vi "MakeWhitePlot.vi"(7 "Canvas":refnum<vi>, 8 "# harmonics":i32=40, 9 "# freq":i32=48, 10 "Bounds":T1, 11 "Complex In":cluster{dbl, "df":dbl, cdb[]}[](array[cluster])) -> (3 "Graph":picture)   [LabVIEW 2022 SP3]
uses:
  <vilib>/Utility/miscctls.llb/LVBoundsTypeDef.ctl
  Perspective/subs/Perspective_Globals.vi
panel:
  out "TRF":cluster{dbl, "df":dbl, dbl[]}(graph)={199.951171875, "df"=0.732421875, array[13381 elements]}
  out "2D Plot":dbl[][](graph)=[[nan, 20.049987226429913, 25.054902961250857, 29.445158043811198, 34.46385501795731, 44.780627225419565, 51.406191185965646, 49.67631609372249, 40.709611963732584, 38.92269108407762, 40.35029451326228, 33.055745098571954, 41.52467260523725, 39.21617102292643, 15.173302135246772, 40.695109109084115, 42.444899082336, 56.77593405896198, 51.382201329207334, 43.21477455890306, 50.80370011373546, 35.98612449368547, 47.77204513443894, 30.857881410259274, 46.643671439889445, 47.49403661581599, -1.4346363375750995, 19.0211768965106, 45.28695989710588, 40.69907700152897, 46.376353342172045, 39.045432783467874, 48.20425730785347, 35.99159002094946, 35.20324613314526, 51.91563451765467, 18.854037759092634, 37.28439063047342, -19.57168106597702, 25.22610299025189, 29.263013635587455, 30.82063676591259, 33.55395737125039, 18.19981181386353, 24.102157288646847, 39.34971755858826, 22.241809662116708, 68.52224965159985], [54.26627490024298, 47.12526752661166, 56.85500723817575, 36.55833093424573, 38.634265924869595, 51.93988341853376, 45.638032395871505, 66.45923338856223, 48.341086236955675, 44.73549896684294, 82.8746731094306, 36.13504669577988, 32.4985458705831, 38.46882120330299, 25.627379738354886, 38.640118352136994, 69.51016913200667, 47.08441844740895, 43.538098543664844, 37.74770538349388, 2.607749244145145, 35.43065545900197, 48.78584596653637, 44.50117153673708, 47.18149466094815, 37.167565780443084, -11.290057999008061, 38.82305284871714, 34.622338104545236, 45.77689163136356, 27.988762535569126, 35.05040002787151, 46.39143083402964, 41.744798474139316, 32.89651926775419, 62.34466322011301, 39.44356696797309, 46.6442728756223, -10.828073640077598, 26.81232522566393, 48.71727144928745, 32.03610040569839, 72.79095309960253, 36.67913423432094, 48.058266713190754, nan, nan, nan], [53.04185758812355, 84.71388448770111, 17.51080377410179, 40.44091855599027, 39.91331658353087, 28.362665427675545, 55.229556863313356, 56.42371074485528, 47.76931799964777, 39.97049168305633, 57.15726261780386, 37.542352295940155, 44.21162796738528, 17.48325982608004, 40.43782874904303, 38.742739205630784, 46.032627402046785, 20.05630274646011, 45.78665416858822, 35.24520049827762, 39.158716639789034, 11.924005690223789, 29.897529283546916, 33.60264045829483, 31.392790303731708, 19.506700819440113, -9.215795080095525, 50.42813350565264, 32.59479614372741, 31.01757424069985, 42.71237559822864, 51.983617982184924, 34.35731157695301, 42.627623260331376, 19.10147623463881, 54.50616438544329, 18.296402637224976, 58.61753732987064, nan, nan, nan, nan, nan, nan, nan, nan, nan, nan], [39.51596652723599, 29.184271442763787, 16.957827346664814, 37.67653983236719, 63.59782300125275, 48.322834414258296, 40.39060448678149, 38.07851466585304, 52.219678596166396, 61.51482106592874, 46.8634576004301, 37.06553982367735, 38.09179565041872, 11.208063972191031, 54.731123202538576, 29.039234290370757, 34.051601948841004, 41.1260225901982, 52.08899147984912, 28.05180790327435, 34.07973803463468, 42.3996411700281, 20.192703080247497, 56.168607595418976, 33.25620455392025, 39.61259618090587, 1.6416847986202243, 24.841476380656804, 37.55245428572219, 27.459839855335257, 66.77063240632266, 36.5729389128255, 41.814287416945945, nan, nan, nan, nan, nan, nan, nan, nan, nan, nan, nan, nan, nan, nan, nan], [48.16850062624863, 42.24542108686359, 44.340073178907026, 3.901363084528417, 42.347676492963295, 41.98102702804944, 32.095730941153256, 7.619084984059836, 32.35066397625168, 32.29142786493228, 40.21124807070387, 14.63732432854075, 64.87319042636963, 3.8937001997797758, 42.35230450100133, 14.130476829463692, 28.642057668910525, 38.68345012614008, 40.520552066845205, 52.826865227382584, 27.4036034714791, 73.37393650330726, 10.947826509906172, 39.440434175724384, 31.785624530969287, 39.726239419396016, 27.00365963632292, 17.381561857680012, 36.93147689751727, nan, nan, nan, nan, nan, nan, nan, nan, nan, nan, nan, nan, nan, nan, nan, nan, nan, nan, nan], [35.60423156346238, 46.08009523979531, 36.87411957248013, 43.245886090198724, 41.3473179130062, 26.344792341973875, 41.08933756077456, 27.303763144444684, 32.28100773510765, 34.38861713258833, 31.00322874795537, 55.966772111396814, 33.80384369988236, 22.921989435884473, 8.945740357752978, 42.39269732229077, 33.87217699897191, 33.14532562541018, 33.524294370197566, 44.041506495823185, 37.757502066680686, 41.939614181516674, 8.546073278104322, 48.000016608061514, 35.00765134648421, 51.85386377302325, nan, nan, nan, nan, nan, nan, nan, nan, nan, nan, nan, nan, nan, nan, nan, nan, nan, nan, nan, nan, nan, nan], [32.61310636745673, 38.97527846530624, 35.641622198785086, 36.36206724043218, 27.795949148894337, 54.187637574190326, 36.401734072540044, 30.917571343879366, 37.20179247250486, 27.793291744454113, 25.775060428523826, 10.666225801452157, 38.49962709844564, 11.781027471364073, 13.761017548356374, 42.53126220573978, 35.128829087408405, 40.161072813389424, 41.09343386515138, 35.9780075897034, 17.001024691654287, 42.92404272966259, 26.64675831650957, nan, nan, nan, nan, nan, nan, nan, nan, nan, nan, nan, nan, nan, nan, nan, nan, nan, nan, nan, nan, nan, nan, nan, nan, nan], [29.681571025848356, 42.60929144128346, 48.67052729500847, 58.6607561868737, 33.95354038216709, 41.11614535668331, 47.65431912163869, -11.009770350280277, 36.94947500875874, 39.83841719056124, 31.381560080516877, 52.500057048302736, 38.174458325750436, 20.80842003831775, 12.283677007960899, 35.16227099829001, 59.770944975043896, 21.937359659167246, 60.53209358540707, 36.682904986845664, 39.7581113435772, nan, nan, nan, nan, nan, nan, nan, nan, nan, nan, nan, nan, nan, nan, nan, nan, nan, nan, nan, nan, nan, nan, nan, nan, nan, nan, nan], [40.464054607466934, 37.58597485171173, 39.87038706581357, 51.19267039727471, 37.67639985297179, 23.13937723997912, 37.55595835553924, 42.4209222579333, 42.27910760517511, 30.522265980669758, 26.136408931304445, -2.9872106006803496, 31.322538117444275, 2.9044348449634656, 3.5797530867064515, 50.092277015634636, 38.50977087060315, 47.533818499292835, 35.62939006713031, nan, nan, nan, nan, nan, nan, nan, nan, nan, nan, nan, nan, nan, nan, nan, nan, nan, nan, nan, nan, nan, nan, nan, nan, nan, nan, nan, nan, nan], [58.5659239452997, 26.982848813621306, 36.31906856692317, 16.66678219935681, 49.49109923197512, 40.11411668922503, 37.75341628139453, 48.30992190831356, 49.081010121114915, 61.181425385472934, 22.430170217674966, 48.6155340973561, 32.675460627661636, 13.916675441379617, 21.021585447450946, 49.25166283256742, 62.27105544588605, nan, nan, nan, nan, nan, nan, nan, nan, nan, nan, nan, nan, nan, nan, nan, nan, nan, nan, nan, nan, nan, nan, nan, nan, nan, nan, nan, nan, nan, nan, nan], [54.412382522142494, 36.137207842053776, 2.764148858981666, 46.372145605984485, 37.243085887419376, 34.537737023825855, 55.257207308976035, 51.464533050016435, 39.80085824725523, 44.11810710124637, 34.10663843132296, 5.979096794947166, 25.782557120064702, 30.561510305365577, 40.94721364933057, nan, nan, nan, nan, nan, nan, nan, nan, nan, nan, nan, nan, nan, nan, nan, nan, nan, nan, nan, nan, nan, nan, nan, nan, nan, nan, nan, nan, nan, nan, nan, nan, nan], [31.369910198236113, 37.07152928092298, 10.648427094010238, 40.65058675099788, 23.51231403437172, 27.206691169768323, 36.277462506216686, 34.08022467450811, 35.763375497264654, 29.232268970303785, 23.380681094116376, 44.186129447967446, 35.05238954844841, 50.27126063942963, nan, nan, nan, nan, nan, nan, nan, nan, nan, nan, nan, nan, nan, nan, nan, nan, nan, nan, nan, nan, nan, nan, nan, nan, nan, nan, nan, nan, nan, nan, nan, nan, nan, nan], [47.82026138668182, 33.43812207351204, 25.299758140785883, -0.1217403502671347, 22.16453525325594, 48.48725544404082, 42.08447575914906, 19.62567783478579, 38.80170108501365, 40.192102073325636, 33.03273363219364, 36.03429599678489, 28.409628306750335, nan, nan, nan, nan, nan, nan, nan, nan, nan, nan, nan, nan, nan, nan, nan, nan, nan, nan, nan, nan, nan, nan, nan, nan, nan, nan, nan, nan, nan, nan, nan, nan, nan, nan, nan], [38.74276193034642, 51.348432885653914, 32.25091267120466, 38.33577783712102, 29.752691953524675, 38.079351040376174, 38.87949376223, 0.26530157389657355, 29.509618670886084, 40.33082643082275, 34.24093489901787, nan, nan, nan, nan, nan, nan, nan, nan, nan, nan, nan, nan, nan, nan, nan, nan, nan, nan, nan, nan, nan, nan, nan, nan, nan, nan, nan, nan, nan, nan, nan, nan, nan, nan, nan, nan, nan], [38.005167377161804, 31.69088276912158, 52.845640027356204, 35.852538445709634, 43.1225994596063, 37.243651148967345, 29.029508255433182, 9.006139857266586, 38.32944523498376, 36.834360308878054, nan, nan, nan, nan, nan, nan, nan, nan, nan, nan, nan, nan, nan, nan, nan, nan, nan, nan, nan, nan, nan, nan, nan, nan, nan, nan, nan, nan, nan, nan, nan, nan, nan, nan, nan, nan, nan, nan], [35.90269660816785, 39.364578709379494, 39.55419749173399, 29.35326642077404, 53.69867614237862, 31.967502560639367, 54.7193336975603, 30.88778141801589, 39.34981484445568, nan, nan, nan, nan, nan, nan, nan, nan, nan, nan, nan, nan, nan, nan, nan, nan, nan, nan, nan, nan, nan, nan, nan, nan, nan, nan, nan, nan, nan, nan, nan, nan, nan, nan, nan, nan, nan, nan, nan], [36.30638411087302, 25.09057920682725, 45.46164717529554, 49.768103526439276, 23.289405968677816, 49.15198590837125, 35.1560324577208, 42.864683043159424, nan, nan, nan, nan, nan, nan, nan, nan, nan, nan, nan, nan, nan, nan, nan, nan, nan, nan, nan, nan, nan, nan, nan, nan, nan, nan, nan, nan, nan, nan, nan, nan, nan, nan, nan, nan, nan, nan, nan, nan], [31.462436582201292, 30.362788351721534, 36.81834627839507, 44.09040502089316, 33.57068005060175, 32.74557557265104, 39.515790233414656, nan, nan, nan, nan, nan, nan, nan, nan, nan, nan, nan, nan, nan, nan, nan, nan, nan, nan, nan, nan, nan, nan, nan, nan, nan, nan, nan, nan, nan, nan, nan, nan, nan, nan, nan, nan, nan, nan, nan, nan, nan], [34.58411077100862, 33.23559013285732, -5.662822029697699, 26.44794576028672, 35.487431815874324, 40.942138140629154, nan, nan, nan, nan, nan, nan, nan, nan, nan, nan, nan, nan, nan, nan, nan, nan, nan, nan, nan, nan, nan, nan, nan, nan, nan, nan, nan, nan, nan, nan, nan, nan, nan, nan, nan, nan, nan, nan, nan, nan, nan, nan], [34.61465926871371, 17.18392844569568, 13.031570274998831, 43.78480234185166, 56.1573881112846, nan, nan, nan, nan, nan, nan, nan, nan, nan, nan, nan, nan, nan, nan, nan, nan, nan, nan, nan, nan, nan, nan, nan, nan, nan, nan, nan, nan, nan, nan, nan, nan, nan, nan, nan, nan, nan, nan, nan, nan, nan, nan, nan], [29.186029345513607, 47.978737915500574, 17.360000383750858, 12.786831883362723, nan, nan, nan, nan, nan, nan, nan, nan, nan, nan, nan, nan, nan, nan, nan, nan, nan, nan, nan, nan, nan, nan, nan, nan, nan, nan, nan, nan, nan, nan, nan, nan, nan, nan, nan, nan, nan, nan, nan, nan, nan, nan, nan, nan], [25.72159338389789, 36.84666611970028, 34.76691669928632, nan, nan, nan, nan, nan, nan, nan, nan, nan, nan, nan, nan, nan, nan, nan, nan, nan, nan, nan, nan, nan, nan, nan, nan, nan, nan, nan, nan, nan, nan, nan, nan, nan, nan, nan, nan, nan, nan, nan, nan, nan, nan, nan, nan, nan], [27.424976418713154, 38.48369817799687, 50.658137928834435, nan, nan, nan, nan, nan, nan, nan, nan, nan, nan, nan, nan, nan, nan, nan, nan, nan, nan, nan, nan, nan, nan, nan, nan, nan, nan, nan, nan, nan, nan, nan, nan, nan, nan, nan, nan, nan, nan, nan, nan, nan, nan, nan, nan, nan], [34.75082504002703, 44.286747839093266, nan, nan, nan, nan, nan, nan, nan, nan, nan, nan, nan, nan, nan, nan, nan, nan, nan, nan, nan, nan, nan, nan, nan, nan, nan, nan, nan, nan, nan, nan, nan, nan, nan, nan, nan, nan, nan, nan, nan, nan, nan, nan, nan, nan, nan, nan], [35.40073024186071, nan, nan, nan, nan, nan, nan, nan, nan, nan, nan, nan, nan, nan, nan, nan, nan, nan, nan, nan, nan, nan, nan, nan, nan, nan, nan, nan, nan, nan, nan, nan, nan, nan, nan, nan, nan, nan, nan, nan, nan, nan, nan, nan, nan, nan, nan, nan], [28.955349958389448, nan, nan, nan, nan, nan, nan, nan, nan, nan, nan, nan, nan, nan, nan, nan, nan, nan, nan, nan, nan, nan, nan, nan, nan, nan, nan, nan, nan, nan, nan, nan, nan, nan, nan, nan, nan, nan, nan, nan, nan, nan, nan, nan, nan, nan, nan, nan], [nan, nan, nan, nan, nan, nan, nan, nan, nan, nan, nan, nan, nan, nan, nan, nan, nan, nan, nan, nan, nan, nan, nan, nan, nan, nan, nan, nan, nan, nan, nan, nan, nan, nan, nan, nan, nan, nan, nan, nan, nan, nan, nan, nan, nan, nan, nan, nan], [nan, nan, nan, nan, nan, nan, nan, nan, nan, nan, nan, nan, nan, nan, nan, nan, nan, nan, nan, nan, nan, nan, nan, nan, nan, nan, nan, nan, nan, nan, nan, nan, nan, nan, nan, nan, nan, nan, nan, nan, nan, nan, nan, nan, nan, nan, nan, nan], [nan, nan, nan, nan, nan, nan, nan, nan, nan, nan, nan, nan, nan, nan, nan, nan, nan, nan, nan, nan, nan, nan, nan, nan, nan, nan, nan, nan, nan, nan, nan, nan, nan, nan, nan, nan, nan, nan, nan, nan, nan, nan, nan, nan, nan, nan, nan, nan], [nan, nan, nan, nan, nan, nan, nan, nan, nan, nan, nan, nan, nan, nan, nan, nan, nan, nan, nan, nan, nan, nan, nan, nan, nan, nan, nan, nan, nan, nan, nan, nan, nan, nan, nan, nan, nan, nan, nan, nan, nan, nan, nan, nan, nan, nan, nan, nan], [nan, nan, nan, nan, nan, nan, nan, nan, nan, nan, nan, nan, nan, nan, nan, nan, nan, nan, nan, nan, nan, nan, nan, nan, nan, nan, nan, nan, nan, nan, nan, nan, nan, nan, nan, nan, nan, nan, nan, nan, nan, nan, nan, nan, nan, nan, nan, nan], [nan, nan, nan, nan, nan, nan, nan, nan, nan, nan, nan, nan, nan, nan, nan, nan, nan, nan, nan, nan, nan, nan, nan, nan, nan, nan, nan, nan, nan, nan, nan, nan, nan, nan, nan, nan, nan, nan, nan, nan, nan, nan, nan, nan, nan, nan, nan, nan], [nan, nan, nan, nan, nan, nan, nan, nan, nan, nan, nan, nan, nan, nan, nan, nan, nan, nan, nan, nan, nan, nan, nan, nan, nan, nan, nan, nan, nan, nan, nan, nan, nan, nan, nan, nan, nan, nan, nan, nan, nan, nan, nan, nan, nan, nan, nan, nan], [nan, nan, nan, nan, nan, nan, nan, nan, nan, nan, nan, nan, nan, nan, nan, nan, nan, nan, nan, nan, nan, nan, nan, nan, nan, nan, nan, nan, nan, nan, nan, nan, nan, nan, nan, nan, nan, nan, nan, nan, nan, nan, nan, nan, nan, nan, nan, nan], [nan, nan, nan, nan, nan, nan, nan, nan, nan, nan, nan, nan, nan, nan, nan, nan, nan, nan, nan, nan, nan, nan, nan, nan, nan, nan, nan, nan, nan, nan, nan, nan, nan, nan, nan, nan, nan, nan, nan, nan, nan, nan, nan, nan, nan, nan, nan, nan], [nan, nan, nan, nan, nan, nan, nan, nan, nan, nan, nan, nan, nan, nan, nan, nan, nan, nan, nan, nan, nan, nan, nan, nan, nan, nan, nan, nan, nan, nan, nan, nan, nan, nan, nan, nan, nan, nan, nan, nan, nan, nan, nan, nan, nan, nan, nan, nan], [nan, nan, nan, nan, nan, nan, nan, nan, nan, nan, nan, nan, nan, nan, nan, nan, nan, nan, nan, nan, nan, nan, nan, nan, nan, nan, nan, nan, nan, nan, nan, nan, nan, nan, nan, nan, nan, nan, nan, nan, nan, nan, nan, nan, nan, nan, nan, nan], [nan, nan, nan, nan, nan, nan, nan, nan, nan, nan, nan, nan, nan, nan, nan, nan, nan, nan, nan, nan, nan, nan, nan, nan, nan, nan, nan, nan, nan, nan, nan, nan, nan, nan, nan, nan, nan, nan, nan, nan, nan, nan, nan, nan, nan, nan, nan, nan], [nan, nan, nan, nan, nan, nan, nan, nan, nan, nan, nan, nan, nan, nan, nan, nan, nan, nan, nan, nan, nan, nan, nan, nan, nan, nan, nan, nan, nan, nan, nan, nan, nan, nan, nan, nan, nan, nan, nan, nan, nan, nan, nan, nan, nan, nan, nan, nan], [nan, nan, nan, nan, nan, nan, nan, nan, nan, nan, nan, nan, nan, nan, nan, nan, nan, nan, nan, nan, nan, nan, nan, nan, nan, nan, nan, nan, nan, nan, nan, nan, nan, nan, nan, nan, nan, nan, nan, nan, nan, nan, nan, nan, nan, nan, nan, nan]]
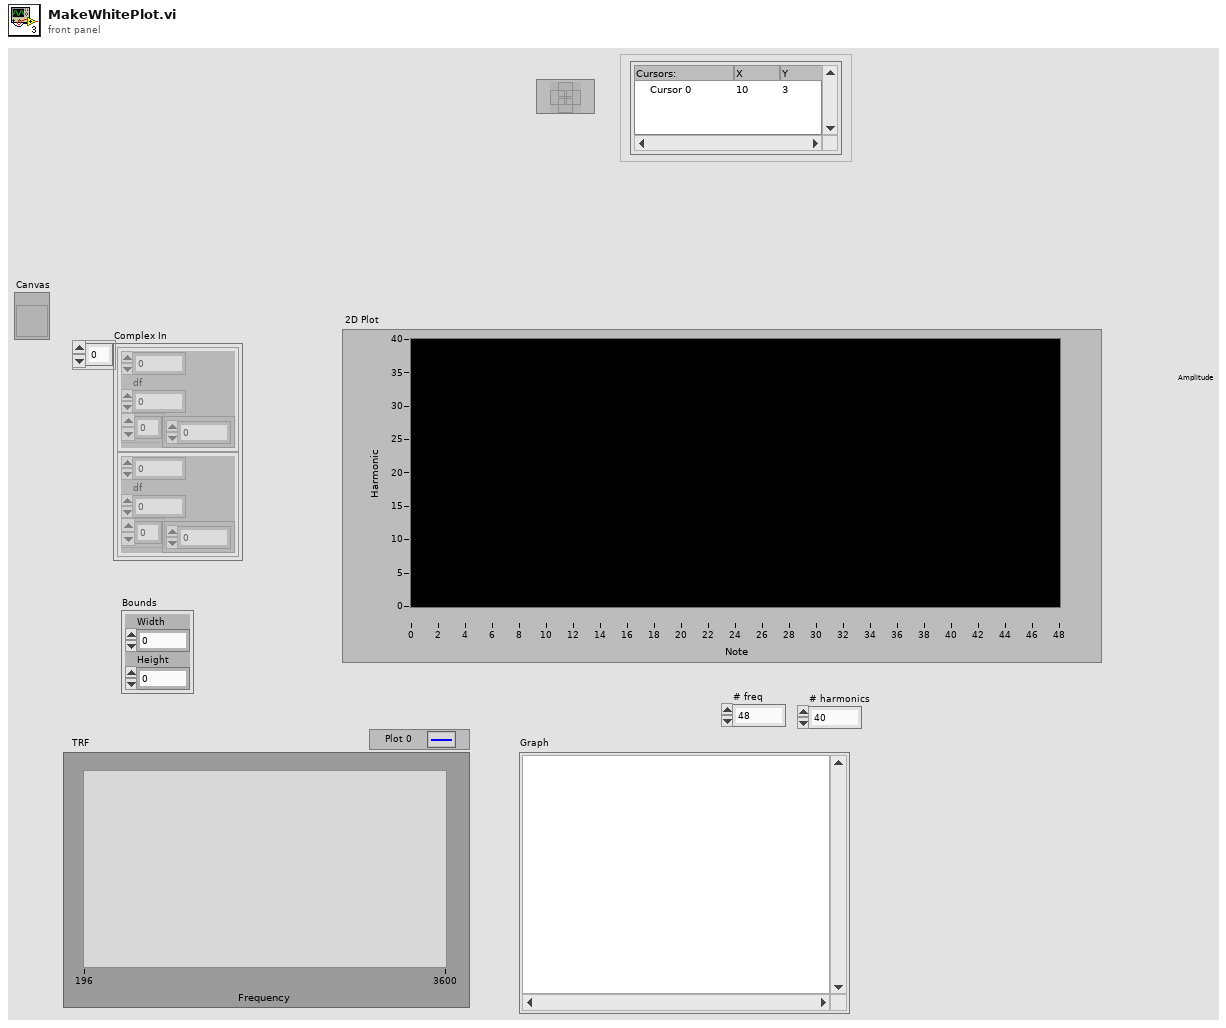
[diagram p1: front panel]
types:
  T1 = typedef "LVBoundsTypeDef.ctl" = cluster{"Width":u32, "Height":u32}
  T2 = enum16{"Sine Wave", "Triangle Wave", "Square Wave", "Sawtooth Wave"}
  T3 = cluster{"Notes":string, "format string":string}[]
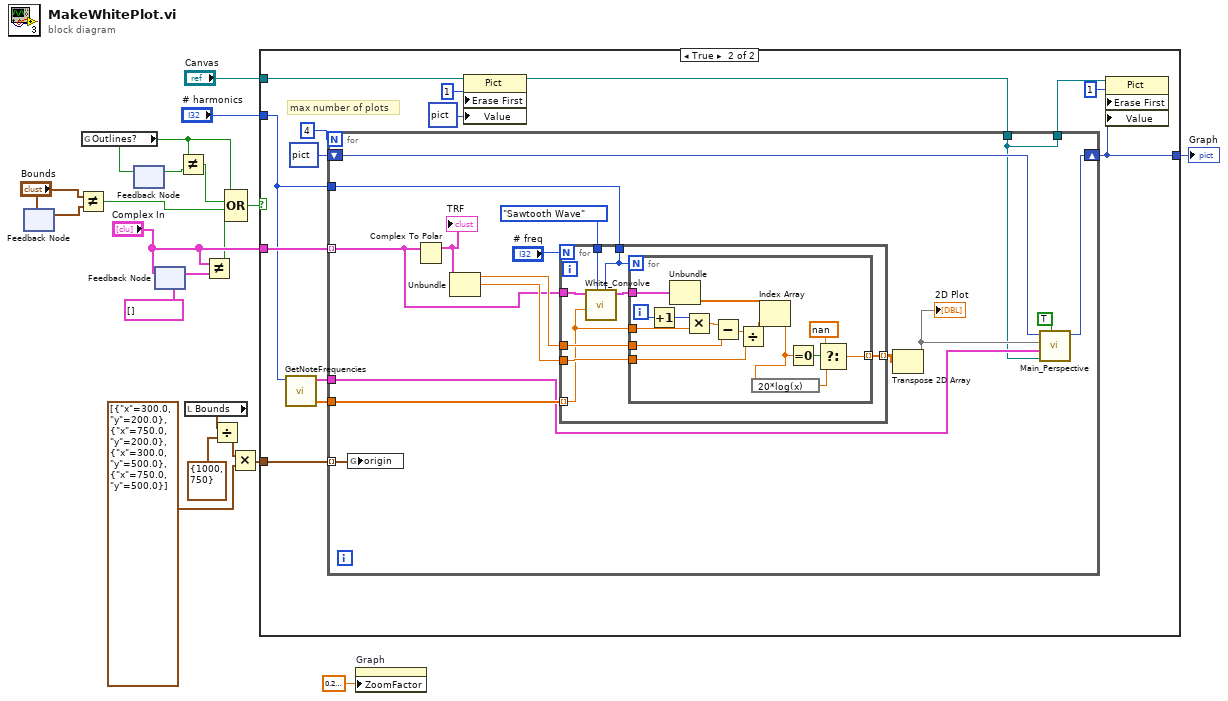
[diagram p0: block diagram]
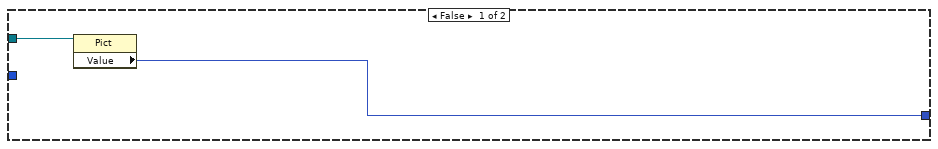
[diagram p2: hidden frame]
diagram:
  n1 = feedback #1() -> (w14:T1)  [unwired: 1 in]
  n2 = feedback-in #1("Bounds") -> ()
  n3 = Not Equal?(x="Bounds", y=w14) -> (x != y?=w13:bool)
  n4 = global read "Perspective_Globals.vi" "Outlines?"() -> (w2:bool)
  n5 = feedback #2() -> (w3:bool)  [unwired: 1 in]
  n6 = feedback-in #2(w2) -> ()
  n7 = feedback-in #3("Complex In") -> ()
  n8 = feedback #3(cluster{dbl, "df":dbl, cdb[]}[] [] ("Complex In")) -> (w16:cluster{dbl, "df":dbl, cdb[]}[])
  n9 = Not Equal?(x=w2, y=w3) -> (x != y?=w1:bool)
  n10 = local read "Bounds"() -> (w4:T1)
  n11 = Not Equal?(x="Complex In", y=w16) -> (x != y?=w12:bool)
  n12 = Divide(x=w4, y=T1 {"Width"=1000, "Height"=750} ("Bounds")) -> (x/y=w7:cluster{"Width":dbl, "Height":dbl})
  n13 = Compound Arithmetic op=OR(w2, w1, w13, w12) -> (w11:bool)
  n14 = Multiply(x=w7, y=cluster{"x":dbl, "y":dbl}[] [{"x"=300.0, "y"=200.0}, {"x"=750.0, "y"=200.0}, {"x"=300.0, "y"=500.0}, {"x"=750.0, "y"=500.0}]) -> (x*y=w5:cluster{dbl, dbl}[])
  n15 = case shown="True" w11 {
    tunnel: "# harmonics" -> [_ w31]
    tunnel: "Complex In" -> [_ w35]
    tunnel: w5 -> [_ w32]
    tunnel: [w21 w27] -> w19
    tunnel: "Canvas" -> [w22 w24]
    frame False {
      n16 = property class="Pict"(reference=w22) -> ("Value"=w21:picture)  [unwired: 1 in, 2 out]
    }
    frame True {
      # "max number of plots"
      n17 = call "GetNoteFrequencies.vi"("# harmonics"=w31) -> ("frequencies"=w34:dbl[], "Labels"=w33:T3)  [unwired: 8 in, 1 out]
      n18 = for {
        N: 4 -> [_]
        tunnel: w31 -> [w44]
        tunnel: w35 -> [w41] mode=indexing
        tunnel: w34 -> [w43]
        tunnel: w33 -> [w42]
        tunnel: w32 -> [w40] mode=indexing
        shift-right: [w38] -> w27
        shift-left: picture data[5B] ("Graph") -> [w37]
        tunnel: w24 -> [w36]
        tunnel: [w36] -> w29
        n19 = global write "Perspective_Globals.vi" "origin"(w40) -> ()
        n20 = Complex To Polar(r * e^(i*theta)=w41) -> (r=w50:cluster{dbl, "df":dbl, dbl[]})  [unwired: 1 out]
        "TRF" <- w50
        n21 = Unbundle(w50) -> (w51:dbl, "df"=w47:dbl)  [unwired: 1 out]
        n22 = for {
          N: "# freq" -> [_]
          tunnel: w41 -> [w55]
          tunnel: [w57] -> w48 mode=indexing
          tunnel: w43 -> [w54] mode=indexing
          tunnel: w51 -> [w58]
          tunnel: w47 -> [w59]
          tunnel: w44 -> [w52]
          tunnel: T2."Sawtooth Wave" ("signal type") -> [w53]
          n23 = call "White_Convolve.vi"("# harmonics"=w52, "signal type"=w53, "frequency"=w54, "Complex FRF"=w55) -> ("convolution"=w56:cluster{dbl, "df":dbl, dbl[]})  [unwired: 7 in]
          n24 = for {
            N: w52 -> [_]
            tunnel: w56 -> [w74]
            tunnel: w54 -> [w70]
            tunnel: w58 -> [w69]
            tunnel: w59 -> [w68]
            tunnel: [w64] -> w57 mode=indexing
            i -> [w66]
            n25 = Increment(x=w66) -> (x+1=w73:i32)
            n26 = Unbundle(w74) -> (w60:dbl[])  [unwired: 2 out]
            n27 = Multiply(x=w73, y=w70) -> (x*y=w72:dbl)
            n28 = Subtract(x=w72, y=w69) -> (x-y=w71:dbl)
            n29 = Divide(x=w71, y=w68) -> (x/y=w67:dbl)
            n30 = Index Array(array=w60, index=w67) -> (element=w62:dbl)
            n31 = expression code="20*log(x)"(w62) -> (w61:dbl)
            n32 = Equal To 0?(x=w62) -> (x = 0?=w65:bool)
            n33 = Select(t=nan, s=w65, f=w61) -> (s? t:f=w64:dbl)
          }
        }
        n34 = Transpose 2D Array(2D array=w48) -> (transposed array=w39:dbl[][])
        "2D Plot" <- w39
        n35 = call "Main_Perspective.vi"("3D?"=TRUE, "reference"=w36, "labels"=w42, "White Plot"=w39, "picture in"=w37) -> ("Graph"=w38:picture)  [unwired: 6 in]
      }
      n36 = property class="Pict"(reference=w24, "Erase First"=u8 1, "Value"=picture data[5B] ("Graph")) -> ()  [unwired: 1 in, 2 out]
      n37 = property class="Pict"(reference=w29, "Erase First"=u8 1, "Value"=w27) -> ()  [unwired: 1 in, 2 out]
    }
  }
  "Graph" <- w19
  n38 = property on="Graph" class="Pict"("ZoomFactor"=sgl 0.2 ("Zoom Factor")) -> ()  [unwired: 2 in, 2 out]
